vi "Set SBOM Component Information.vi"(8 "error in (no error)":errorcluster, 10 "CycloneDX Component":refnum<class "CycloneDX Component.lvclass">, 11 "CycloneDX SBOM in":refnum<class "CycloneDX SBOM.lvclass">) -> (0 "error out":errorcluster, 3 "CycloneDX SBOM out":refnum<class "CycloneDX SBOM.lvclass">)   [LabVIEW 2017, in "LabVIEW CycloneDX SBOM.lvlib" / "CycloneDX SBOM.lvclass"]
doc: "Set the metadata component information of the overall SBOM. This describes the component that the SBOM has been created for."
uses:
  CycloneDX SBOM.lvclass
  C:/LabVIEW Working Directory/labview-cyclonedx-sbom/Source/CycloneDX/CycloneDX JSON/CycloneDX JSON.lvclass
  CycloneDX Component/CycloneDX Component.lvclass
  CycloneDX JSON/CycloneDX JSON.lvclass/CycloneDX JSON.ctl
  CycloneDX JSON/Read JSON.vi
  CycloneDX JSON/CycloneDX JSON.lvclass
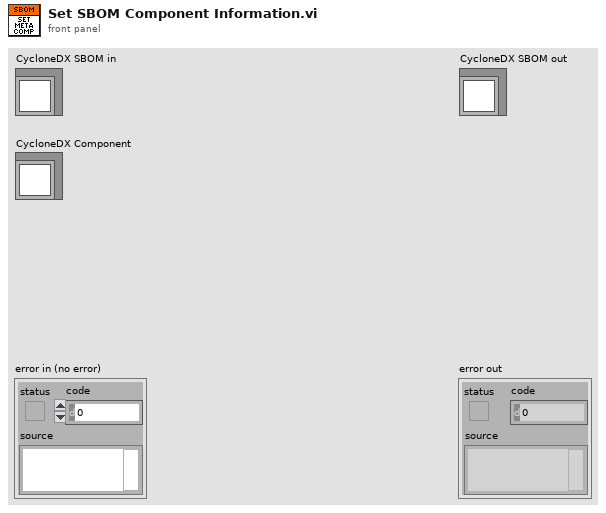
[diagram p1: front panel]
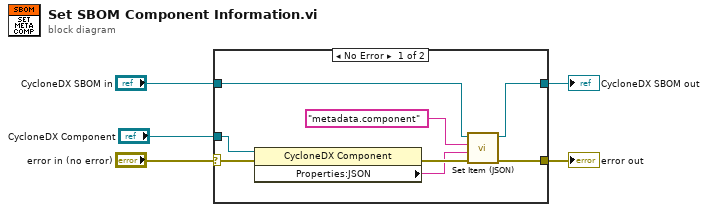
[diagram p0: block diagram]
diagram:
  n1 = case shown="No Error" "error in (no error)" {
    selector: "error in (no error)" -> [w9 w15]
    tunnel: [w11 w15] -> w4
    tunnel: [w12 w14] -> w2
    tunnel: "CycloneDX SBOM in" -> [w13 w14]
    tunnel: "CycloneDX Component" -> [w10 _]
    frame No Error {
      n2 = property class="CycloneDX Component"(reference=w10, error in=w9) -> (error out=w7:errorcluster, "Properties:JSON"=w6:string)  [unwired: 1 out]
      n3 = call "Set Item (JSON).vi"("error in (no error)"=w7, "JSON to Insert"=w6, "Object (or Item) Path"="metadata.component", "CycloneDX SBOM in"=w13) -> ("error out"=w11:errorcluster, "CycloneDX SBOM out"=w12:refnum<class "CycloneDX SBOM.lvclass">)  [unwired: 6 in]
    }
    frame Error {
    }
  }
  "error out" <- w4
  "CycloneDX SBOM out" <- w2
